vi "Configure Tag Voltage Pulse.vi"   [LabVIEW 2017, in "Keithley 2600 Series.lvlib"]
doc: "Configures a pulsed voltage sweep with a current measurement."
uses:
  <instrlib>/Keithley 2600 Series/Keithley 2600 Series.lvlib
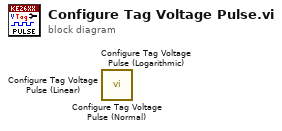
[diagram p0: block diagram]
diagram:
  n1 = call <instrlib>:"Configure Tag Voltage Pulse (Normal).vi"() -> ()  [unwired: 26 in, 2 out]
  n2 = call <instrlib>:"Configure Tag Voltage Pulse (Logarithmic).vi"() -> ()  [unwired: 26 in, 2 out]
  n3 = call <instrlib>:"Configure Tag Voltage Pulse (Linear).vi"() -> ()  [unwired: 26 in, 2 out]
